vi "Hold for Fetch.vi"(8 "error in (no error)":errorcluster, 10 "Hold for Fetch (T: Enable)":bool=TRUE, 11 "VISA resource name":refnum<visa-resource-name>) -> (0 "error out":errorcluster, 3 "VISA resource name out":refnum<visa-resource-name>)   [LabVIEW 2021, in "Yokogawa WT1800 Series.lvlib"]
doc: "Sets the hold/release status of the waveform data hold feature for all waveforms.\nAs long as <b>Hold for Fetch</b> is enable, waveform data is held even when the\nwaveform display on the screen is updated."
uses:
  <instrlib>/Yokogawa WT1800 Series/Yokogawa WT1800 Series.lvlib
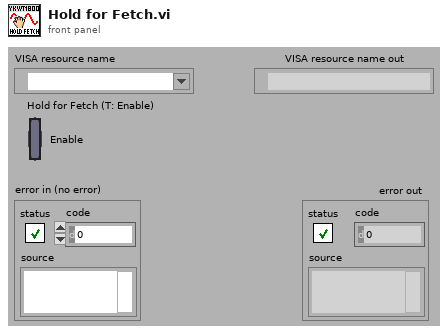
[diagram p1: front panel]
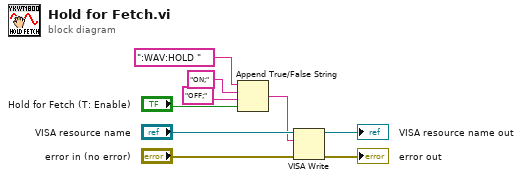
[diagram p0: block diagram]
diagram:
  n1 = Append True/False String ("True/False 文字列を追加")(1:"Hold for Fetch (T: Enable)", 2:"OFF;", 3:"ON;", 4:":WAV:HOLD ") -> (0:w1:string)
  n2 = VISA Write ("VISA書き込み")(VISA resource name="VISA resource name", write buffer=w1, error in (no error)="error in (no error)") -> (VISA resource name out=→"VISA resource name out":refnum<visa-resource-name>, error out=→"error out":errorcluster)  [unwired: 1 out]
